vi "Fire Set Timeout User Event.vi"(8 "error in (no error)":errorcluster, 10 "Timeout":i32, 11 "Wait User Events":T1) -> (0 "error out":errorcluster)   [LabVIEW 2023, in "Weather Wait Loop.lvlib"]
doc: "Generates the wait message loop's set timeout user event to modify the event loop's timeout duration."
uses:
  Weather Wait Loop.lvlib
  User Events.ctl
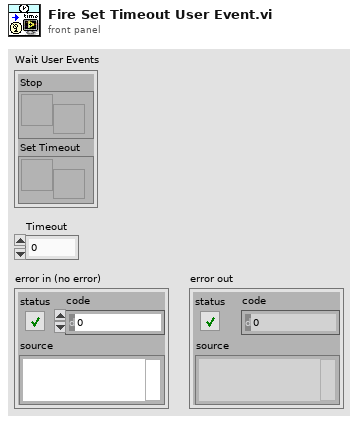
[diagram p1: front panel]
types:
  T1 = typedef "Weather Wait Loop.lvlib/User Events.ctl" = cluster{"Stop":refnum<user-event>, "Set Timeout":refnum<user-event>}
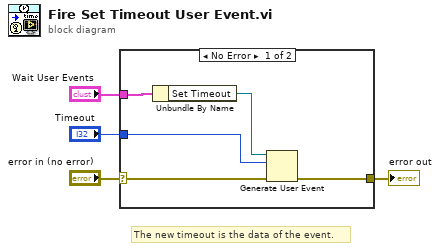
[diagram p0: block diagram]
diagram:
  # "The new timeout is the data of the event."
  n1 = case shown="No Error" "error in (no error)" {
    selector: "error in (no error)" -> [w9 w10]
    tunnel: [w8 w10] -> w3
    tunnel: "Wait User Events" -> [w7 _]
    tunnel: "Timeout" -> [w5 _]
    frame No Error {
      n2 = Unbundle By Name(w7) -> ("Set Timeout"=w6:refnum<user-event>)
      n3 = Generate User Event(user event=w6, event data cluster=w5, error in=w9) -> (error out=w8:errorcluster)  [unwired: 1 in, 1 out]
    }
    frame Error {
    }
  }
  "error out" <- w3
